vi "NI-USB-6210_Kernel.vi"() -> (0 "error out":errorcluster)   [LabVIEW 2013]
uses:
  <vilib>/DAQmx/read.llb/DAQmx Read (Analog 2D DBL NChan NSamp).vi
  Globals/measurementGlobal.vi
  <vilib>/DAQmx/configure/timing.llb/DAQmx Timing (Sample Clock).vi
  <vilib>/DAQmx/create/channels.llb/DAQmx Create Channel (AI-Voltage-Basic).vi
  <vilib>/DAQmx/miscellaneous.llb/DAQmx Fill In Error Info.vi
panel:
  out "Block Index":i32
  out "Case":string[](array[string])
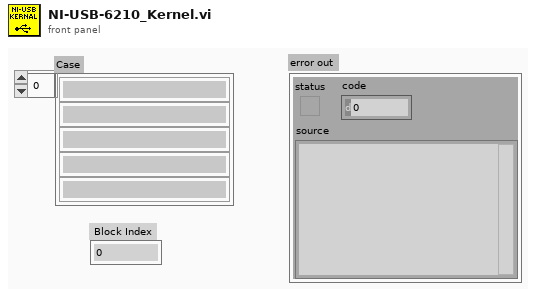
[diagram p1: front panel]
types:
  T1 = cluster{"Chan No.":i32, "Low Volt Limit (-10V)":dbl, "High Volt Limit (10V)":dbl, "input terminal configuration":i32}[]
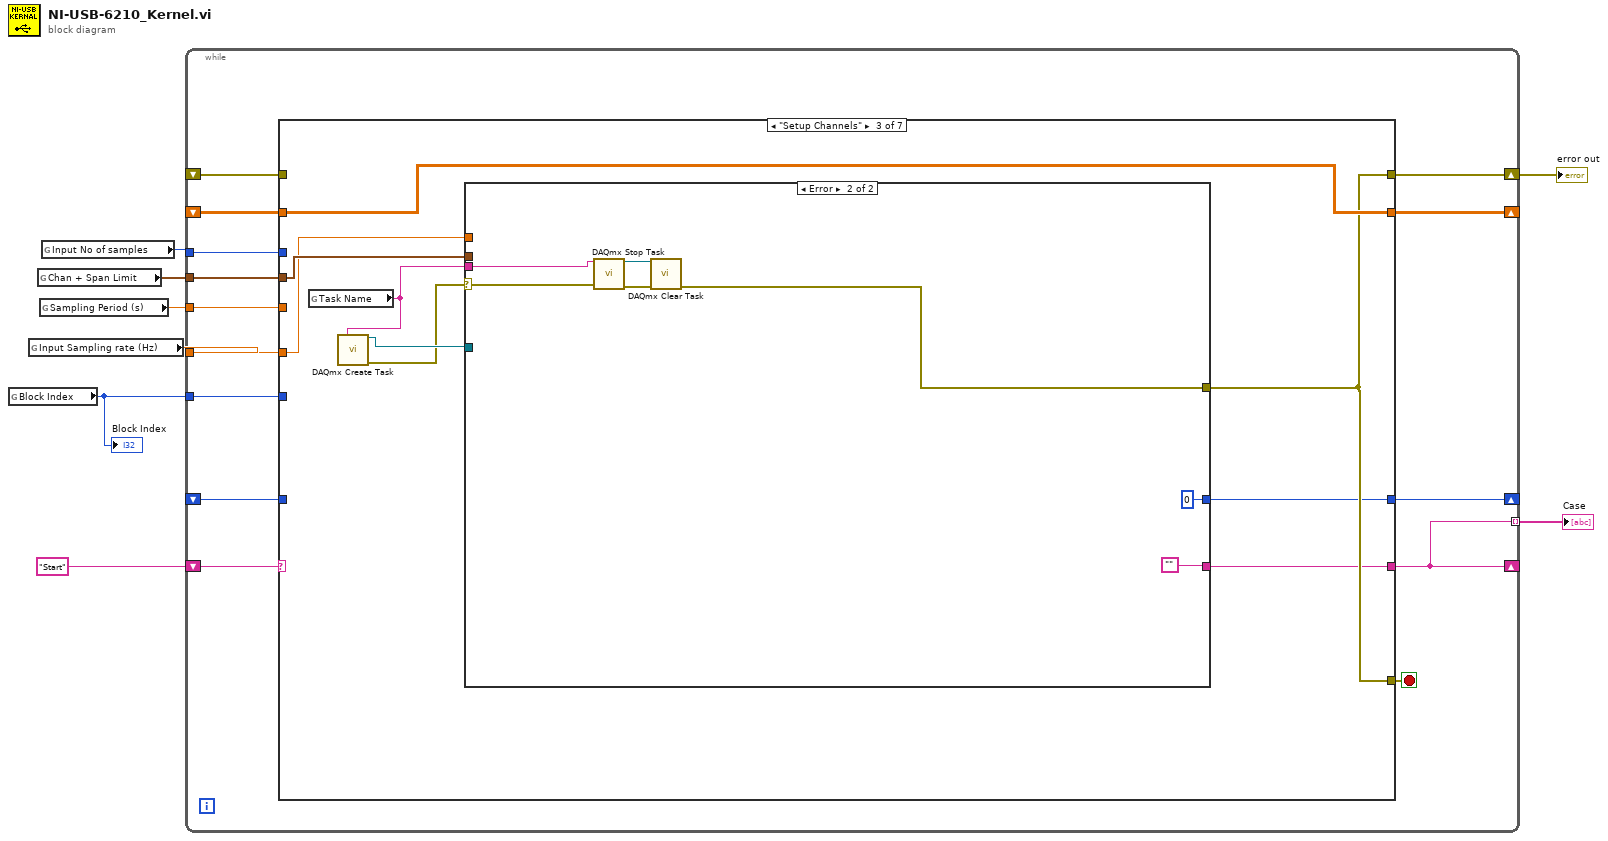
[diagram p0: block diagram]
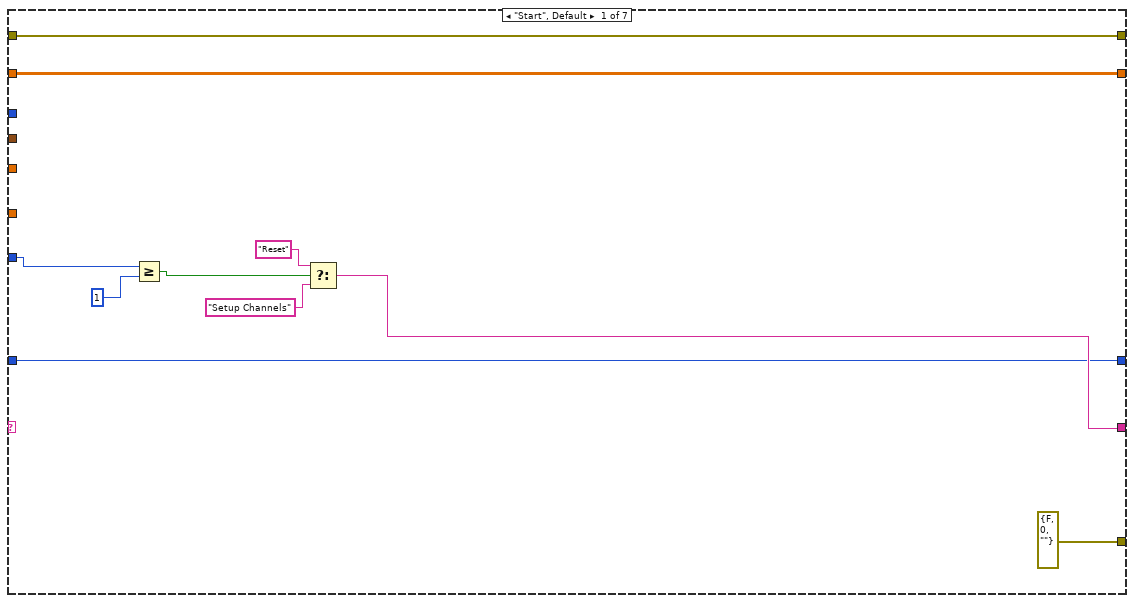
[diagram p2: hidden frame]
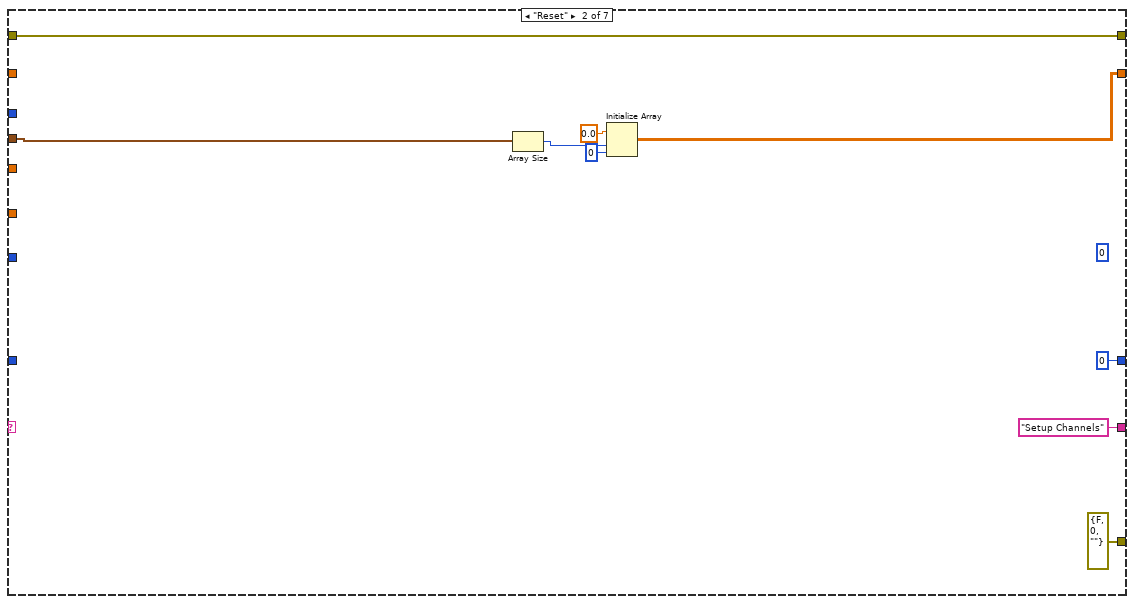
[diagram p3: hidden frame]
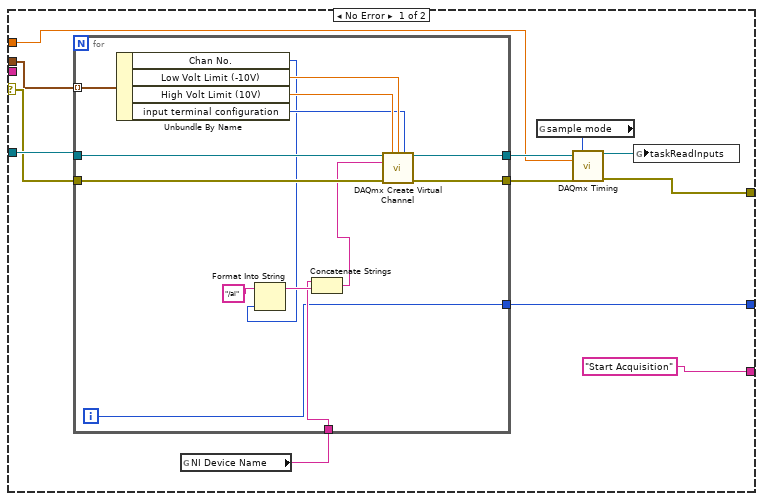
[diagram p4: hidden frame]
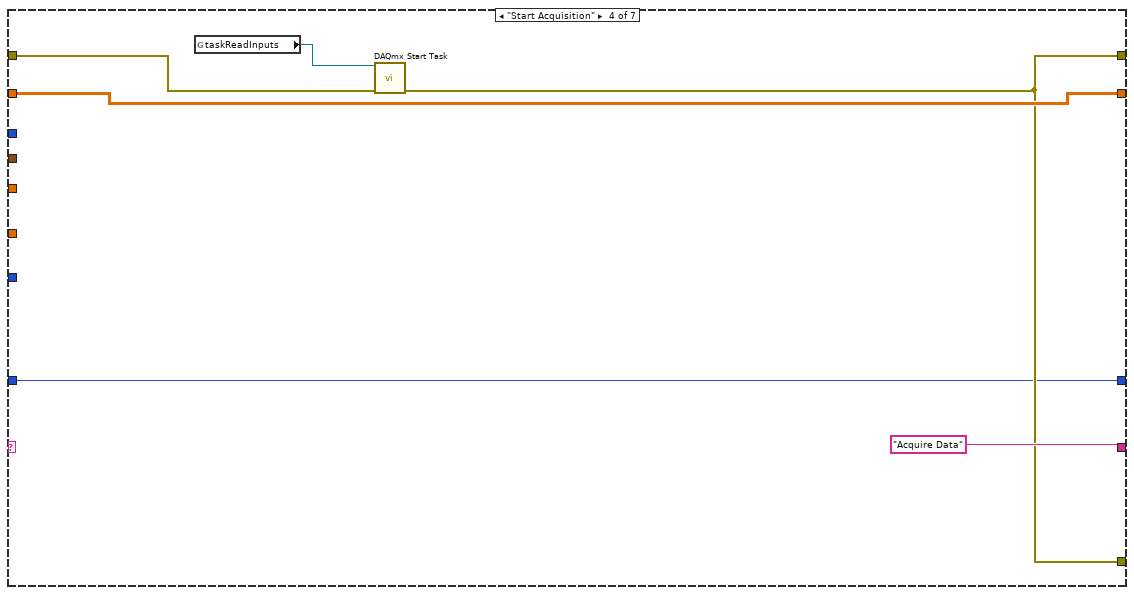
[diagram p5: hidden frame]
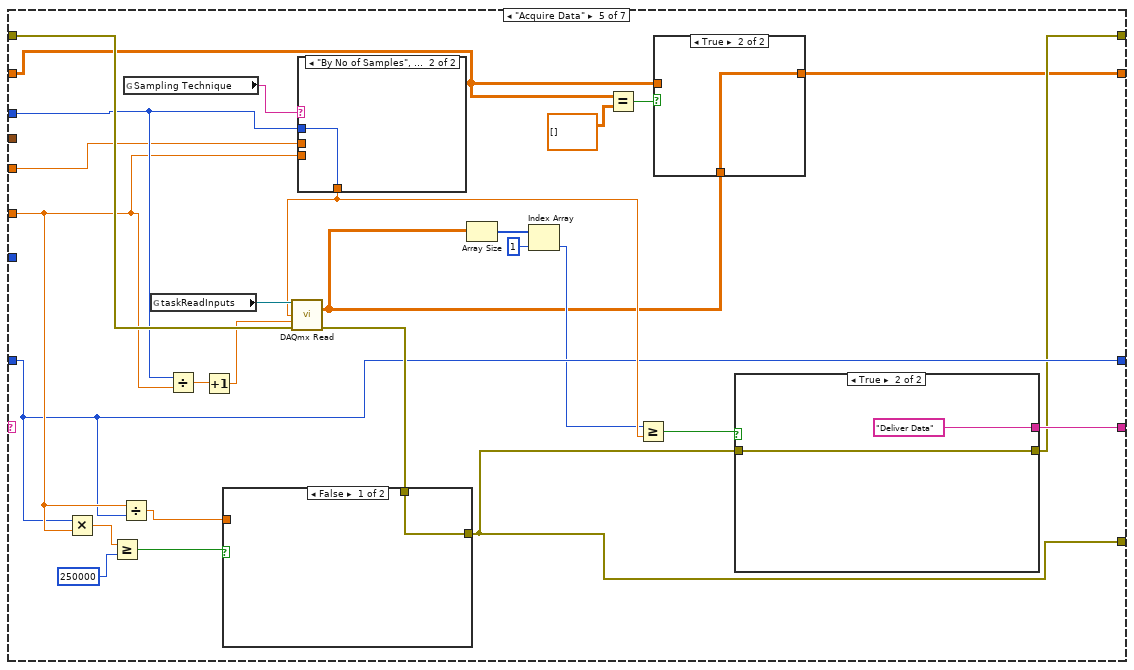
[diagram p6: hidden frame]
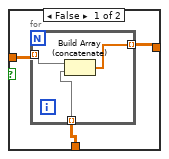
[diagram p7: hidden frame]
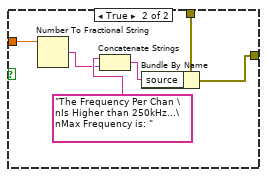
[diagram p8: hidden frame]
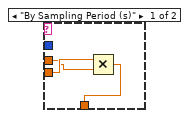
[diagram p9: hidden frame]
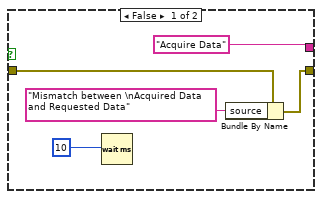
[diagram p10: hidden frame]
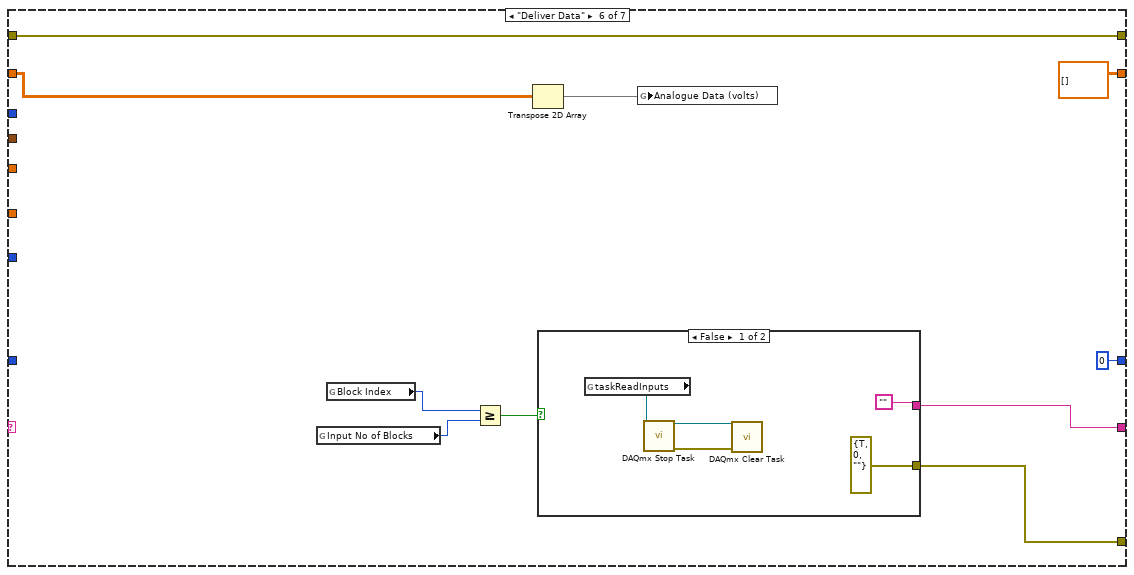
[diagram p11: hidden frame]
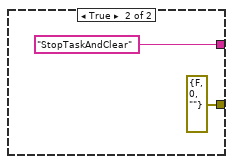
[diagram p12: hidden frame]
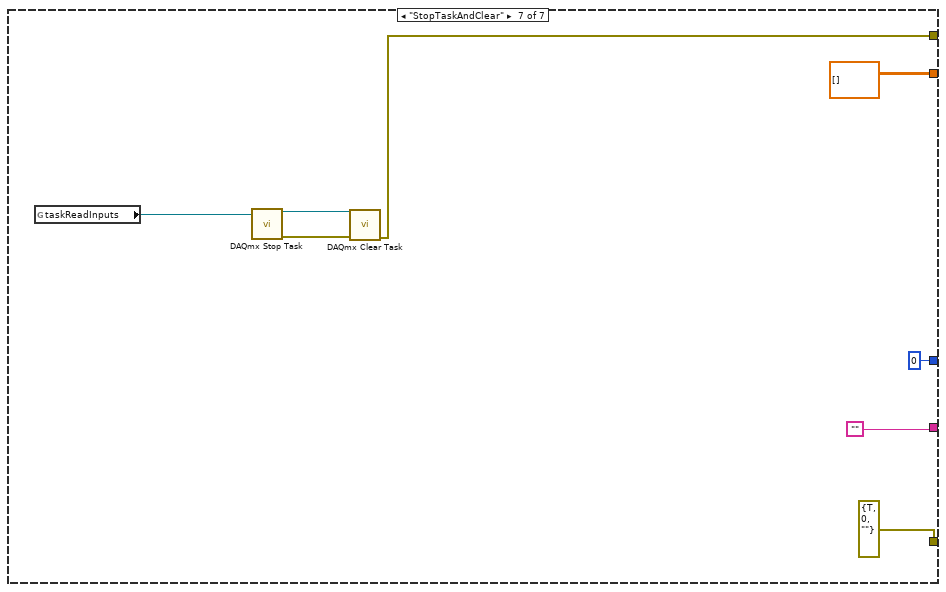
[diagram p13: hidden frame]
diagram:
  n1 = global read "measurementGlobal.vi" "Block Index"() -> (w1:i32)
  "Block Index" <- w1
  n2 = global read "measurementGlobal.vi" "Input Sampling rate (Hz)"() -> (w7:dbl)
  n3 = global read "measurementGlobal.vi" "Chan + Span Limit"() -> (w3:T1)
  n4 = global read "measurementGlobal.vi" "Sampling Period (s)"() -> (w2:dbl)
  n5 = global read "measurementGlobal.vi" "Input No of samples"() -> (w8:i32)
  n6 = while {
    tunnel: w8 -> [w22]
    tunnel: w7 -> [w21]
    shift-right: [w20] -> w6
    shift-left: _ -> [w19]
    shift-right: [w13] -> _
    shift-left: _ -> [w17]
    shift-right: [w15] -> _
    shift-left: "Start" -> [w16]
    tunnel: [w15] -> w4 mode=indexing
    tunnel: w3 -> [w14]
    tunnel: w2 -> [w12]
    shift-right: [w10] -> _
    shift-left: _ -> [w11]
    tunnel: w1 -> [w9]
    stop <- w18 stop-if-true
    n7 = case shown="\"Setup Channels\"" w16 {
      tunnel: w22 -> [_ _ _ _ w107 _ _]
      tunnel: w21 -> [_ _ w45 _ w100 _ _]
      tunnel: [w26 w39 w44 w85 w96 w151 w164] -> w20
      tunnel: w19 -> [w26 w39 _ w88 w115 w151 _]
      tunnel: [errorcluster {"status"=FALSE, "code"=0, "source"=""} ("error out") errorcluster {"status"=FALSE, "code"=0, "source"=""} ("error out") w44 w85 w97 w142 errorcluster {"status"=TRUE, "code"=0, "source"=""} ("error out")] -> w18
      tunnel: [w32 w33 w50 w87 w90 dbl[][] [] ("data") dbl[][] [] ("data")] -> w13
      tunnel: w17 -> [w32 _ w50 w87 w91 w145 _]
      tunnel: [w27 "Setup Channels" ("f") w43 "Acquire Data" w111 w148 ""] -> w15
      tunnel: w14 -> [_ w37 w46 _ _ _ _]
      tunnel: w12 -> [_ _ _ _ w106 _ _]
      tunnel: w11 -> [w24 _ _ w84 w99 _ _]
      tunnel: [w24 0 w42 w84 w99 0 0] -> w10
      tunnel: w9 -> [w23 _ _ _ _ _ _]
      frame "Start", Default {
        n8 = Greater Or Equal?(x=w23, y=1) -> (x >= y?=w30:bool)
        n9 = Select(t="Reset", s=w30, f="Setup Channels") -> (s? t:f=w27:string)
      }
      frame "Reset" {
        (unwired) 0 ("Block Index")
        n10 = Array Size(array=w37) -> (size(s)=w36:i32)
        n11 = Initialize Array(0.0 ("element"), w36, 0 ("dimension size")) -> (w33:dbl[][])
      }
      frame "Setup Channels" {
        n12 = global read "measurementGlobal.vi" "Task Name"() -> (w47:string)
        n13 = call <vilib>:"DAQmx Create Task.vi"("new task name"=w47) -> ("task out"=w49:refnum<k21>, "error out"=w48:errorcluster)  [unwired: 13 in]
        n14 = case shown="Error" w48 {
          selector: w48 -> [w60 w80]
          tunnel: w46 -> [w59 _]
          tunnel: w49 -> [w61 _]
          tunnel: w47 -> [_ w82]
          tunnel: [w53 w79] -> w44
          tunnel: w45 -> [w55 _]
          tunnel: ["Start Acquisition" ""] -> w43
          tunnel: [w51 0] -> w42
          frame No Error {
            n15 = global read "measurementGlobal.vi" "NI Device Name"() -> (w62:string)
            n16 = for {
              tunnel: w59 -> [w64] mode=indexing
              tunnel: w62 -> [w70]
              tunnel: [w76] -> w56
              tunnel: [w75] -> w54
              tunnel: w61 -> [w74]
              tunnel: w60 -> [w73]
              tunnel: [w63] -> w51
              i -> [w63]
              n17 = Unbundle By Name(w64) -> ("Chan No."=w65:i32, "Low Volt Limit (-10V)"=w69:dbl, "High Volt Limit (10V)"=w68:dbl, "input terminal configuration"=w67:i32)
              n18 = Format Into String(initial string="/ai", w65) -> (resulting string=w71:string)  [unwired: 2 in, 1 out]
              n19 = Concatenate Strings(w70, w71) -> (w66:string)
              n20 = call-poly <vilib>:"DAQmx Create Virtual Channel.vi"("task in"=w74, "maximum value"=w68, "minimum value"=w69, "input terminal configuration"=w67, "physical channels"=w66, "error in"=w73) -> ("task out"=w76:refnum<k21>, "error out"=w75:errorcluster)  [unwired: 8 in]
            }
            n21 = global read "measurementGlobal.vi" "sample mode"() -> (w58:i32)
            n22 = call-poly <vilib>:"DAQmx Timing.vi"("task/channels in"=w56, "sample mode"=w58, "rate"=w55, "error in"=w54) -> ("task out"=w57:refnum<k21>, "error out"=w53:errorcluster)  [unwired: 10 in]
            n23 = global write "measurementGlobal.vi" "taskReadInputs"(w57) -> ()
          }
          frame Error {
            n24 = call <vilib>:"DAQmx Stop Task.vi"("task/channels in"=w82, "error in"=w80) -> ("task out"=w81:refnum<k21>, "error out"=w83:errorcluster)  [unwired: 12 in]
            n25 = call <vilib>:"DAQmx Clear Task.vi"("task in"=w81, "error in"=w83) -> ("error out"=w79:errorcluster)  [unwired: 13 in]
          }
        }
      }
      frame "Start Acquisition" {
        n26 = global read "measurementGlobal.vi" "taskReadInputs"() -> (w89:refnum<k21>)
        n27 = call <vilib>:"DAQmx Start Task.vi"("task/channels in"=w89, "error in"=w88) -> ("error out"=w85:errorcluster)  [unwired: 12 in, 1 out]
      }
      frame "Acquire Data" {
        n28 = Multiply(x=w99, y=w100) -> (x*y=w104:dbl)
        n29 = Greater Or Equal?(x=w104, y=250000) -> (x >= y?=w102:bool)
        n30 = Divide(x=w100, y=w99) -> (x/y=w98:dbl)
        n31 = global read "measurementGlobal.vi" "Sampling Technique"() -> (w108:string)
        n32 = global read "measurementGlobal.vi" "taskReadInputs"() -> (w110:refnum<k21>)
        n33 = Divide(x=w107, y=w100) -> (x/y=w116:dbl)
        n34 = Increment(x=w116) -> (x+1=w109:dbl)
        n35 = case shown="\"By No of Samples\", Default" w108 {
          tunnel: [w131 w134] -> w105
          tunnel: w107 -> [_ w134]
          tunnel: w100 -> [w133 _]
          tunnel: w106 -> [w132 _]
          frame "By Sampling Period (s)" {
            n36 = Multiply(x=w133, y=w132) -> (x*y=w131:dbl)
          }
          frame "By No of Samples", Default {
          }
        }
        n37 = call-poly <vilib>:"DAQmx Read.vi"("task/channels in"=w110, "number of samples per channel"=w105, "timeout"=w109, "error in"=w115) -> ("data"=w92:dbl[][], "error out"=w101:errorcluster)  [unwired: 9 in, 1 out]
        n38 = case shown="False" w102 {
          tunnel: w101 -> [w124 w130]
          tunnel: [w124 w129] -> w97
          tunnel: w98 -> [_ w128]
          frame False {
          }
          frame True {
            n39 = Number To Fractional String(number=w128) -> (F-format string=w126:string)  [unwired: 3 in]
            n40 = Concatenate Strings("The Frequency Per Chan \nIs Higher than 250kHz...\nMax Frequency is: " ("source"), w126) -> (w125:string)
            n41 = Bundle By Name(cluster=w130, "source"=w125) -> (w129:errorcluster)
          }
        }
        n42 = Array Size(array=w92) -> (size(s)=w114:i32[])
        n43 = Index Array(array=w114, index=1) -> (element=w95:i32)
        n44 = Equal?(x=w91, y=dbl[][] []) -> (x = y?=w94:bool)
        n45 = Greater Or Equal?(x=w95, y=w105) -> (x >= y?=w112:bool)
        n46 = case shown="True" w94 {
          tunnel: w92 -> [w118 w123]
          tunnel: [w117 w123] -> w90
          tunnel: w91 -> [w119 _]
          frame False {
            n47 = for {
              tunnel: w119 -> [w122] mode=indexing
              tunnel: w118 -> [w121] mode=indexing
              tunnel: [w120] -> w117 mode=indexing
              n48 = Build Array (concatenate)(w122, w121) -> (w120:dbl[])
            }
          }
          frame True {
          }
        }
        n49 = case shown="True" w112 {
          tunnel: ["Acquire Data" "Deliver Data"] -> w111
          tunnel: w97 -> [w137 w140]
          tunnel: [w135 w140] -> w96
          frame False {
            n50 = Wait (ms)(milliseconds to wait=u32 10) -> ()  [unwired: 1 out]
            n51 = Bundle By Name(cluster=w137, "source"="Mismatch between \nAcquired Data and Requested Data") -> (w135:errorcluster)
          }
          frame True {
          }
        }
      }
      frame "Deliver Data" {
        n52 = global read "measurementGlobal.vi" "Input No of Blocks"() -> (w150:i32)
        n53 = global read "measurementGlobal.vi" "Block Index"() -> (w143:i32)
        n54 = Greater Or Equal?(x=w143, y=w150) -> (x >= y?=w149:bool)
        n55 = Transpose 2D Array(2D array=w145) -> (transposed array=w144:dbl[][])
        n56 = case shown="False" w149 {
          tunnel: ["" "StopTaskAndClear"] -> w148
          tunnel: [errorcluster {"status"=TRUE, "code"=0, "source"=""} ("error out") errorcluster {"status"=FALSE, "code"=0, "source"=""} ("error out")] -> w142
          frame False {
            n57 = global read "measurementGlobal.vi" "taskReadInputs"() -> (w154:refnum<k21>)
            n58 = call <vilib>:"DAQmx Stop Task.vi"("task/channels in"=w154) -> ("task out"=w152:refnum<k21>, "error out"=w153:errorcluster)  [unwired: 13 in]
            n59 = call <vilib>:"DAQmx Clear Task.vi"("task in"=w152, "error in"=w153) -> ()  [unwired: 13 in, 1 out]
          }
          frame True {
          }
        }
        n60 = global write "measurementGlobal.vi" "Analogue Data (volts)"(w144) -> ()
      }
      frame "StopTaskAndClear" {
        n61 = global read "measurementGlobal.vi" "taskReadInputs"() -> (w166:refnum<k21>)
        n62 = call <vilib>:"DAQmx Stop Task.vi"("task/channels in"=w166) -> ("task out"=w163:refnum<k21>, "error out"=w165:errorcluster)  [unwired: 13 in]
        n63 = call <vilib>:"DAQmx Clear Task.vi"("task in"=w163, "error in"=w165) -> ("error out"=w164:errorcluster)  [unwired: 13 in]
      }
    }
  }
  "error out" <- w6
  "Case" <- w4
